vi "Connect Datastream Port.vi"(8 "error in (no error)":errorcluster, 11 "OXY_SCPI Resource In":string="192.168.0.10") -> (0 "error out":errorcluster, 3 "OXY_SCPI Resource Out":refnum<visa-resource-name>)   [LabVIEW 2020, in "OXYGEN_Datastream.lvlib"]
uses:
  OXYGEN_Datastream.lvlib
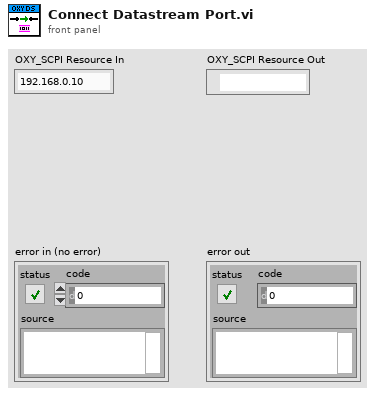
[diagram p1: front panel]
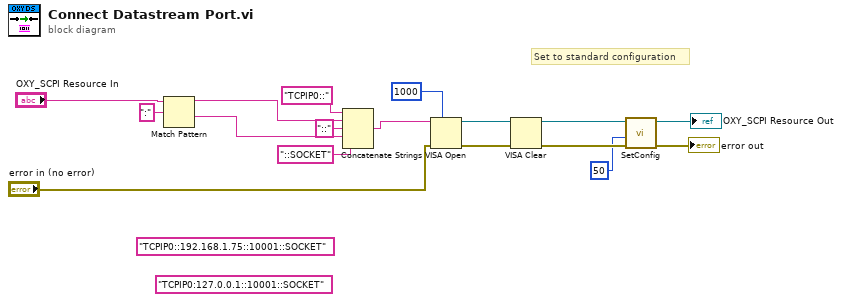
[diagram p0: block diagram]
diagram:
  (unwired) "TCPIP0:127.0.0.1::10001::SOCKET" ("string")
  (unwired) "TCPIP0::192.168.1.75::10001::SOCKET" ("string")
  # "Set to standard configuration"
  n1 = Match Pattern(string="OXY_SCPI Resource In", regular expression=":") -> (before substring=w12:string, after substring=w11:string)  [unwired: 1 in, 2 out]
  n2 = Concatenate Strings("TCPIP0::" ("string"), w12, "::" ("string"), w11, "::SOCKET" ("string")) -> (w8:string)
  n3 = VISA Open(timeout (0)=u32 1000 ("VISA Open timeout (0)"), error in (no error)="error in (no error)", VISA resource name=w8) -> (VISA resource name=w6:refnum<visa-resource-name>, error out=w7:errorcluster)  [unwired: 2 in]
  n4 = VISA Clear(VISA resource name=w6, error in (no error)=w7) -> (VISA resource name out=w5:refnum<visa-resource-name>, error out=w4:errorcluster)
  n5 = call "SetConfig.vi"("error in (no error)"=w4, "Timeout"=u32 50, "OXY_SCPI Reseource In"=w5) -> ("error out"=→"error out":errorcluster, "OXY_SCPI Reseource Out"=→"OXY_SCPI Resource Out":refnum<visa-resource-name>)  [unwired: 7 in]
